vi "Edit Configuration File.vi"() -> ()   [LabVIEW 2017, in "DSF Core.lvlib"]
uses:
  DSF Core.lvlib
  Typedefs/DSF Engine Framework Configuration.ctl
  Typedefs/DSF Engine Plugin Configuration.ctl
  Typedefs/DSF Timing Info.ctl
  Typedefs/DSF Engine Plugin Thread Configuration.ctl
  Typedefs/DSF Settings Info.ctl
  Typedefs/DSF Engine Transfer Group Configuration.ctl
  Typedefs/DSF Direction.ctl
  Typedefs/DSF Engine Transfer Configuration.ctl
  Typedefs/DSF Byte Order.ctl
  Typedefs/DSF Engine Channel Configuration.ctl
  Typedefs/DSF Data Type.ctl
  Typedefs/DSF Timeout Behavior.ctl
  Configuration Session.lvclass
panel:
  out "Duration":dbl format="%.3f s"
  in  "Framework Configuration":T1
  in  "Save":bool
  in  "Load":bool
  in  "Path":path
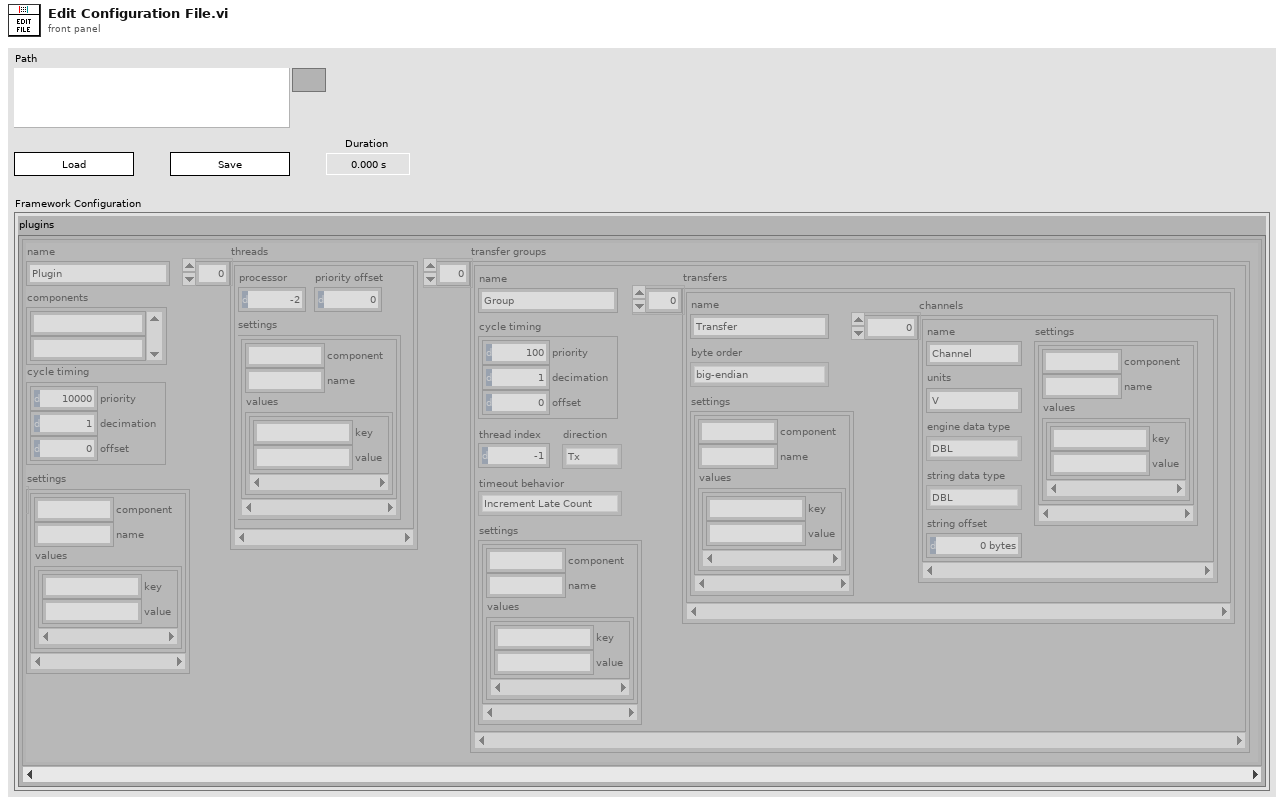
[diagram p1: front panel]
types:
  T1 = typedef "DSF Core.lvlib/DSF Engine Framework Configuration.ctl" = cluster{"plugins":T2[]}
  T2 = typedef "DSF Core.lvlib/DSF Engine Plugin Configuration.ctl" = cluster{"name":string, "components":string[], "cycle timing":T3, "threads":T4[], "transfer groups":T6[], "settings":T5}
  T3 = typedef "DSF Core.lvlib/DSF Timing Info.ctl" = cluster{"priority":u64, "decimation":u64, "offset":u64}
  T4 = typedef "DSF Core.lvlib/DSF Engine Plugin Thread Configuration.ctl" = cluster{"processor":i32, "priority offset":i16, "settings":T5}
  T5 = typedef "DSF Core.lvlib/DSF Settings Info.ctl" = cluster{"component":string, "name":string, "values":cluster{"key":string, "value":string}[]}[]
  T6 = typedef "DSF Core.lvlib/DSF Engine Transfer Group Configuration.ctl" = cluster{"name":string, "direction":T7, "cycle timing":T3, "thread index":i32, "settings":T5, "transfers":T8[], "timeout behavior":T12}
  T7 = typedef "DSF Core.lvlib/DSF Direction.ctl" = enum8{"Tx", "Rx"}
  T8 = typedef "DSF Core.lvlib/DSF Engine Transfer Configuration.ctl" = cluster{"name":string, "byte order":T9, "settings":T5, "channels":T10[]}
  T9 = typedef "DSF Core.lvlib/DSF Byte Order.ctl" = enum8{"big-endian", "little-endian"}
  T10 = typedef "DSF Core.lvlib/DSF Engine Channel Configuration.ctl" = cluster{"string offset":u64, "name":string, "units":string, "engine data type":T11, "string data type":T11, "settings":T5}
  T11 = typedef "DSF Core.lvlib/DSF Data Type.ctl" = enum8{"Bool", "SGL", "DBL", "I8", "I16", "I32", "I64", "U8", "U16", "U32", "U64"}
  T12 = typedef "DSF Core.lvlib/DSF Timeout Behavior.ctl" = enum8{"Increment Late Count", "Throw Error"}
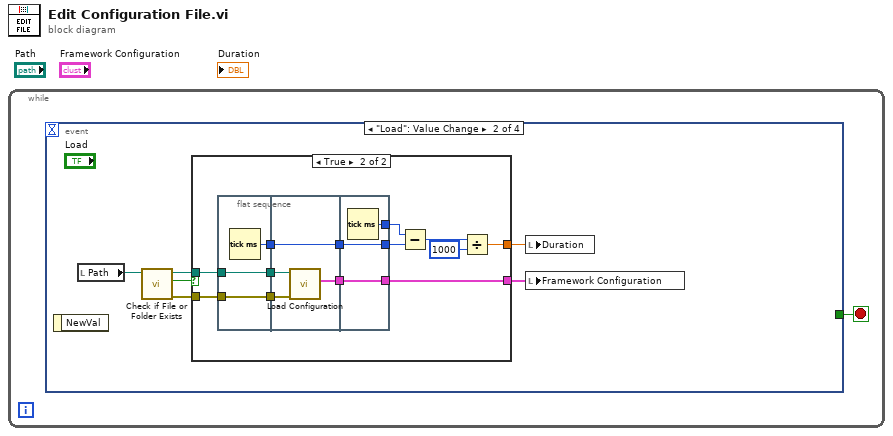
[diagram p0: block diagram]
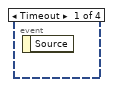
[diagram p2: hidden frame]
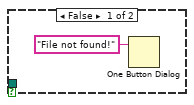
[diagram p3: hidden frame]
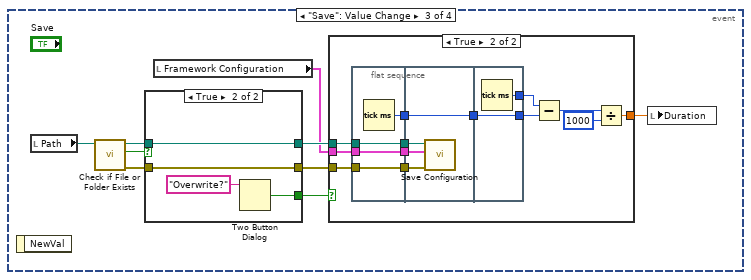
[diagram p4: hidden frame]
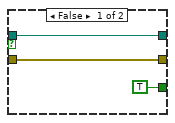
[diagram p6: hidden frame]
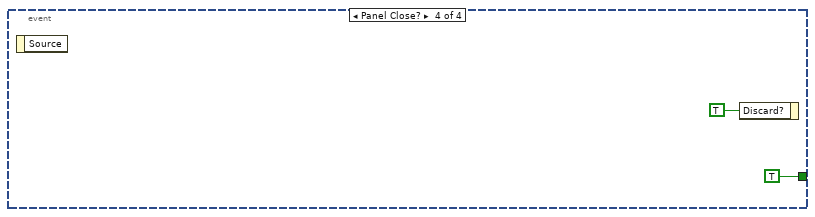
[diagram p7: hidden frame]
diagram:
  n1 = while {
    stop <- w1 stop-if-true
    n2 = event shown="[1] \"Load\": Value Change" {
      selector: _ -> [_ _ _ _]
      dyn-events: _ -> [_ _ _ _]
      timeout: _ -> [_ _ _ _]
      tunnel: [_ _ _ TRUE] -> w1
      event Timeout {
        n3 = event-data() -> ()  [unwired: 1 in, 1 out]
      }
      event "Load": Value Change {
        n4 = event-data() -> ()  [unwired: 1 in, 1 out]
        n5 = local read "Path"() -> (w7:path)
        n6 = call <vilib>:"Check if File or Folder Exists.vi"("path"=w7) -> ("error out"=w6:errorcluster, "file or folder exists?"=w4:bool, "dup path"=w5:path)  [unwired: 8 in]
        n7 = case shown="True" w4 {
          tunnel: w6 -> [_ w21]
          tunnel: w5 -> [_ w20]
          tunnel: [_ w19] -> w3
          tunnel: [_ w9] -> w2
          frame False {
            n8 = One Button Dialog(message="File not found!") -> ()  [unwired: 1 in, 1 out]
          }
          frame True {
            n9 = flat-sequence {
              tunnel: w20 -> [w23]
              tunnel: w21 -> [w24]
              tunnel: [w24] -> w18
              tunnel: [w23] -> w17
              tunnel: [w22] -> w15
              tunnel: w18 -> [w28]
              tunnel: w17 -> [w27]
              tunnel: [w26] -> w16
              tunnel: w15 -> [w25]
              tunnel: [w25] -> w14
              tunnel: [w31] -> w19
              tunnel: w16 -> [w31]
              tunnel: w14 -> [w30]
              tunnel: [w30] -> w13
              tunnel: [w29] -> w12
              frame #0 {
                n10 = Tick Count (ms)() -> (millisecond timer value=w22:u32)
              }
              frame #1 {
                n11 = call "Load Configuration.vi"("error in (no error)"=w28, "configuration file path"=w27) -> ("configuration"=w26:T1)  [unwired: 6 in, 3 out]
              }
              frame #2 {
                n12 = Tick Count (ms)() -> (millisecond timer value=w29:u32)
              }
            }
            n13 = Subtract(x=w12, y=w13) -> (x-y=w11:u32)
            n14 = Divide(x=w11, y=u32 1000) -> (x/y=w9:dbl)
          }
        }
        n15 = local write "Duration"(w2) -> ()
        n16 = local write "Framework Configuration"(w3) -> ()
      }
      event "Save": Value Change {
        n17 = event-data() -> ()  [unwired: 1 in, 1 out]
        n18 = local read "Path"() -> (w40:path)
        n19 = call <vilib>:"Check if File or Folder Exists.vi"("path"=w40) -> ("error out"=w39:errorcluster, "file or folder exists?"=w37:bool, "dup path"=w38:path)  [unwired: 8 in]
        n20 = case shown="True" w37 {
          tunnel: w39 -> [w64 w69]
          tunnel: w38 -> [w65 w67]
          tunnel: [TRUE ("T button?") w68] -> w36
          tunnel: [w65 w67] -> w34
          tunnel: [w64 w69] -> w35
          frame False {
          }
          frame True {
            n21 = Two Button Dialog(message="Overwrite?") -> (T button?=w68:bool)  [unwired: 2 in]
          }
        }
        n22 = local read "Framework Configuration"() -> (w32:T1)
        n23 = case shown="True" w36 {
          tunnel: w35 -> [_ w44]
          tunnel: w34 -> [_ w45]
          tunnel: [_ w43] -> w33
          tunnel: w32 -> [_ w41]
          frame False {
          }
          frame True {
            n24 = flat-sequence {
              tunnel: w45 -> [w56]
              tunnel: w44 -> [w57]
              tunnel: [w57] -> w53
              tunnel: [w56] -> w52
              tunnel: [w55] -> w51
              tunnel: [w54] -> w42
              tunnel: w41 -> [w54]
              tunnel: w53 -> [w59]
              tunnel: w52 -> [w60]
              tunnel: w51 -> [w61]
              tunnel: [w61] -> w50
              tunnel: w42 -> [w58]
              tunnel: w50 -> [w63]
              tunnel: [w63] -> w47
              tunnel: [w62] -> w48
              frame #0 {
                n25 = Tick Count (ms)() -> (millisecond timer value=w55:u32)
              }
              frame #1 {
                n26 = call "Save Configuration.vi"("error in (no error)"=w59, "configuration"=w58, "configuration file path"=w60) -> ()  [unwired: 5 in, 4 out]
              }
              frame #2 {
                n27 = Tick Count (ms)() -> (millisecond timer value=w62:u32)
              }
            }
            n28 = Subtract(x=w48, y=w47) -> (x-y=w49:u32)
            n29 = Divide(x=w49, y=u32 1000) -> (x/y=w43:dbl)
          }
        }
        n30 = local write "Duration"(w33) -> ()
      }
      event Panel Close? {
        n31 = event-data() -> ()  [unwired: 1 in, 1 out]
        n32 = event-data("Discard?"=TRUE) -> ()  [unwired: 1 in, 1 out]
      }
    }
  }
